vi "GetColors.vi"(11 "VGA_data":T1={"x_frontporch"=16, "x_syncpulse"=96, "x_backporch"=48, "y_frontporch"=10, "y_syncpulse"=2, "y_backporch"=33, "DrawPixel?"=FALSE, "x_tickcount"=0, "y_tickcount"=0, "x_Index"=-1, "y_Index"=-1, "x_shift"=0}) -> (2 "Colors":fxp<+,3,3>, 3 "VGA_data 2":T1={"x_frontporch"=16, "x_syncpulse"=96, "x_backporch"=48, "y_frontporch"=10, "y_syncpulse"=2, "y_backporch"=33, "DrawPixel?"=FALSE, "x_tickcount"=0, "y_tickcount"=0, "x_Index"=-1, "y_Index"=-1, "x_shift"=0})   [LabVIEW 2019, in "VGA.lvlib"]
uses:
  VGA.lvlib
  data.ctl
  <vilib>/rvi/Memory/Memory_Emulation/nirvimemoryFastEmulation.vi
  <vilib>/rvi/Memory/Memory_Emulation/nirvimemoryEmulation.vi
  <vilib>/rvi/Emulation/niFpgaEmulationIsFPGAContextNoSignature.vi
  <vilib>/rvi/DataTransferAndStorage/Container/Common/niFpgaContainerGetUniqueNameForEmu.vi
  <vilib>/rvi/Emulation/niFpgaProcessEmulError.vi
  <vilib>/rvi/Emulation/niFpgaSctlEmulationGetInTimedLoop.vi
  <vilib>/rvi/errors/nirviReportUnexpectedCaseInternalError (U32).vi
  <vilib>/rvi/DataTransferAndStorage/Container/XNode/niFpgaContainer.xnode
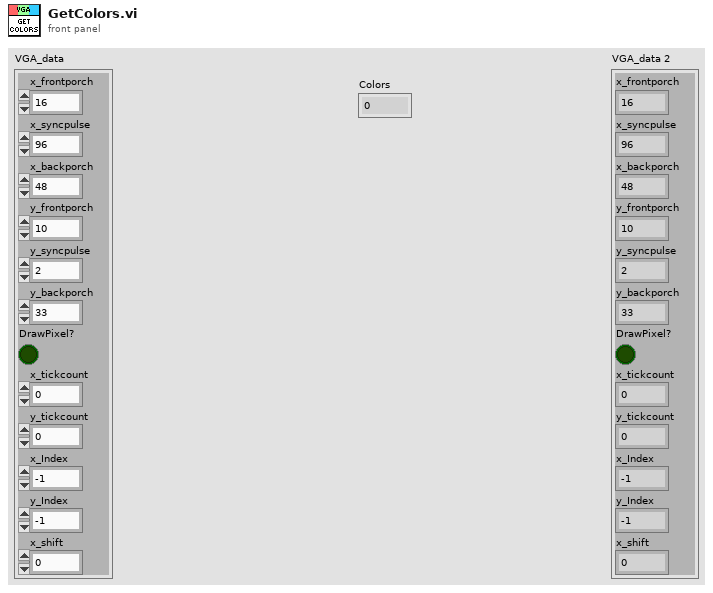
[diagram p1: front panel]
types:
  T1 = typedef "VGA.lvlib/data.ctl" = cluster{"x_frontporch":u8, "x_syncpulse":u8, "x_backporch":u8, "y_frontporch":u8, "y_syncpulse":u8, "y_backporch":u8, "DrawPixel?":bool, "x_tickcount":u16, "y_tickcount":u16, "x_Index":i16, "y_Index":i16, "x_shift":i16}
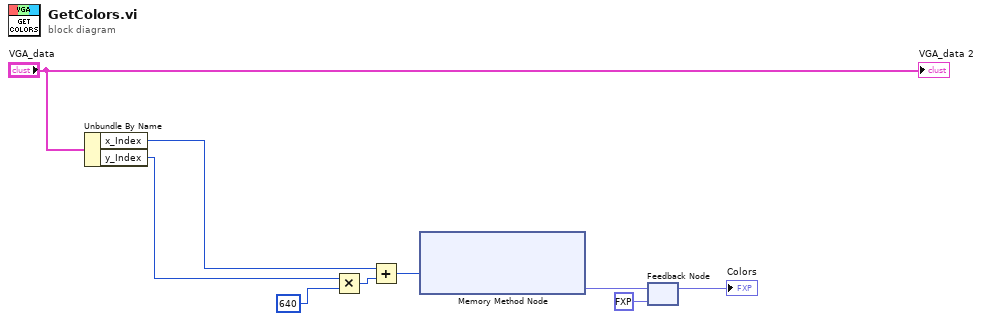
[diagram p0: block diagram]
diagram:
  n1 = Unbundle By Name("VGA_data") -> ("x_Index"=w9:i16, "y_Index"=w8:i16)
  n2 = Multiply(x=w8, y=u16 640 ("Res_Width (640)")) -> (x*y=w3:u32)
  n3 = Add(x=w9, y=w3) -> (x+y=w5:u32)
  n4 = xnode ("Memory Method Node")("Address"=w5) -> ("Data"=w2:fxp<+,3,3>)  [unwired: 1 in, 1 out]
  n5 = feedback #1(fxp<+,3,3> 0.0 ("Data")) -> (→"Colors":fxp<+,3,3>)
  n6 = feedback-in #1(w2) -> ()
  "VGA_data 2" <- "VGA_data"
